vi "Tatica.vi"(9 "InfoMissao":T1 {"Agentes Disponíveis" format="%#_13g"}, 10 "test module 2":T2, 11 "IA State Input 2":T4 {"enemy_robots"."Agentes Disponíveis" format="%#_13g"; "our_robots"."Agentes Disponíveis" format="%#_13g"}) -> (1 "Robot 2":dbl(graph), 2 "ball 2":dbl(graph), 3 "IA State Output 2":T4 {"enemy_robots"."Agentes Disponíveis" format="%#_13g"; "our_robots"."Agentes Disponíveis" format="%#_13g"})   [LabVIEW 2018]
uses:
  Core/AI Input.ctl
  Core/AI Robot.ctl
  Intel/Functions Enum.ctl
  Intel/AttackerStates.ctl
  Path Planning/RRT/PathDests.ctl
  Path Planning/RRT/PathDest.ctl
  Core/AI Ball.ctl
  Core/Field Size.ctl
  Core/AI Judge.ctl
  Intel/Command Enum.ctl
  Util/Events/Events.ctl
  Test/TestModule.ctl
  Util/Select None or Robot.ctl
  InfoMissao.ctl
  <vilib>/Analysis/_algsub.llb/Real Vector Norm.vi
  <vilib>/Analysis/NI_AALPro.lvlib
panel:
  in  "test module":T2
  out "ball":dbl(graph)
  in  "atacando ao contrário?":bool=TRUE
  out "IA State Output":T4 {"enemy_robots"."Agentes Disponíveis" format="%#_13g"; "our_robots"."Agentes Disponíveis" format="%#_13g"}
  in  "IA State Input":T4 {"enemy_robots"."Agentes Disponíveis" format="%#_13g"; "our_robots"."Agentes Disponíveis" format="%#_13g"}
  out "Robot":dbl(graph)
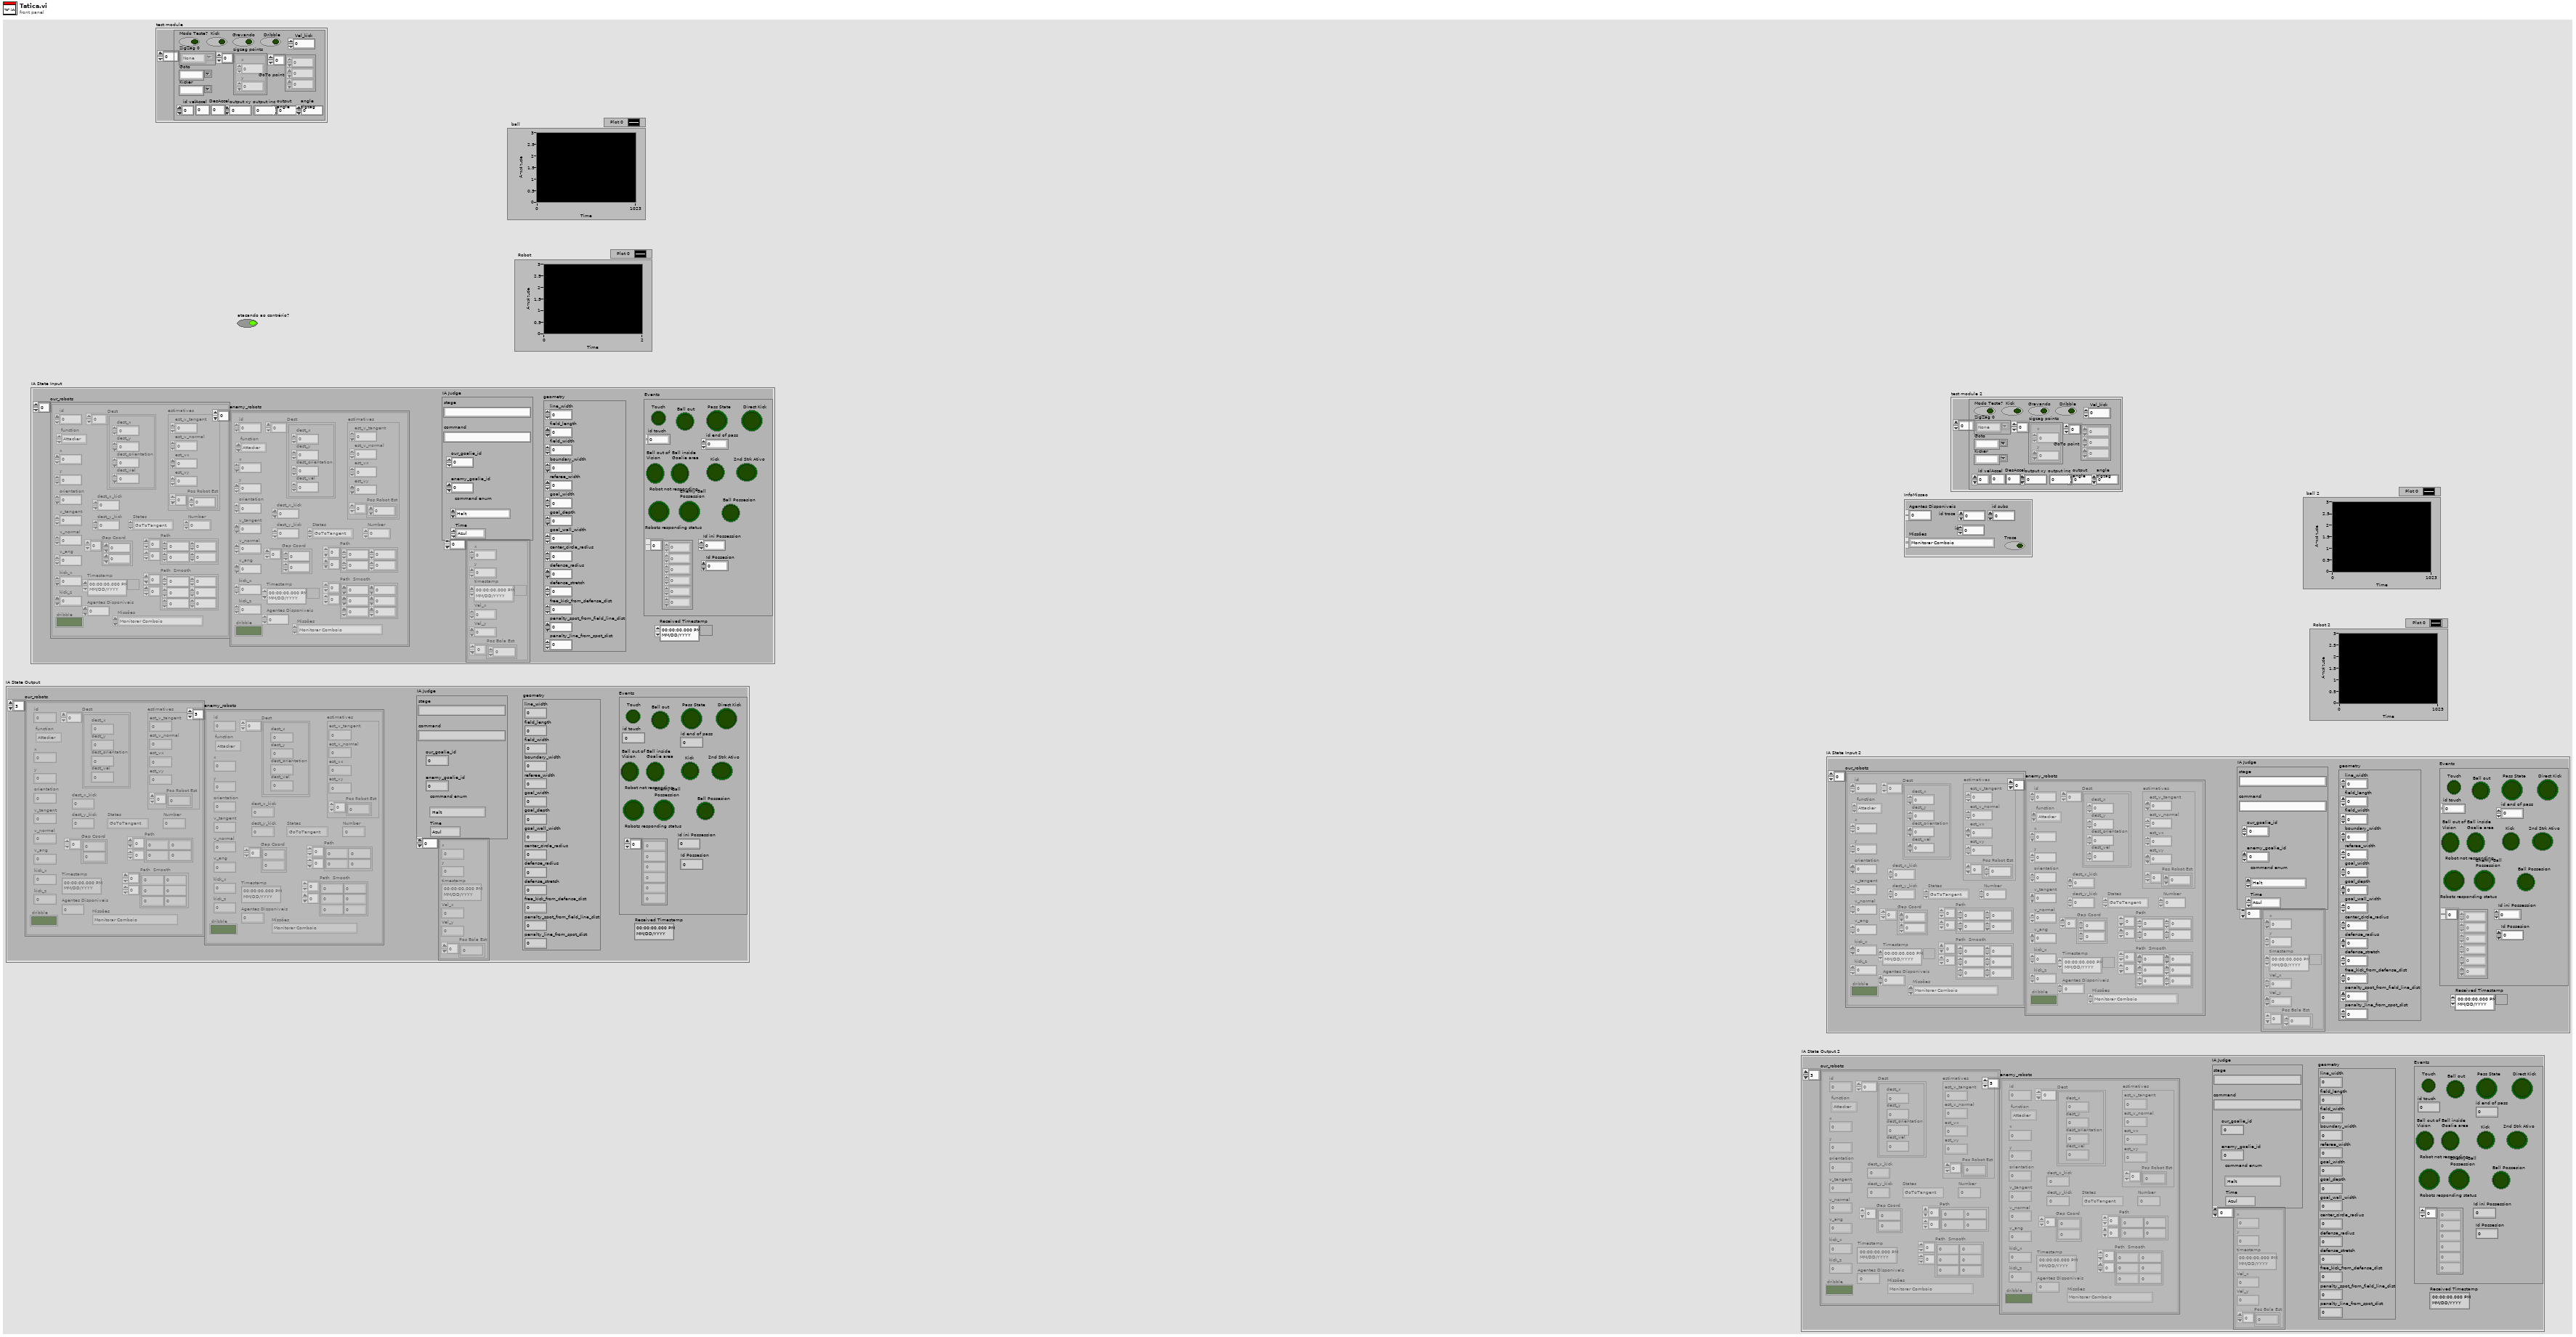
[diagram p1: front panel]
types:
  T1 = typedef "InfoMissao.ctl" = cluster{"Troca ":bool, "Missões ":enum16{"Monitorar Comboio", "Realizar Segurança de Retaguarda", "Vigiar Área", "Reconhecimento de Área"}, "Agentes Disponíveis":dbl, "id troca ":dbl, "id subs":dbl, "id ":dbl}
  T2 = typedef "TestModule.ctl" = cluster{"Goto":T3, "ZigZag 0":T3[], "Kicker":T3, "Vel_kick":dbl, "Kick":bool, "Modo Teste?":bool, "GoTo point":dbl[], "zigzag points":cluster{"x":dbl, "y":dbl}[], " id vel":u32, "Dribble":bool, "Gravando":bool, "output xy":dbl, "output\nangle":dbl, "angle\nzigzag":dbl, "output inc":dbl, "Accel":dbl, "DesAccel":dbl}
  T3 = typedef "Select None or Robot.ctl" = string
  T4 = typedef "AI Input.ctl" = cluster{"our_robots":T5[], "enemy_robots":T5[], "balls":T10[], "geometry":T11, "IA Judge":T12, "Received Timestamp":timestamp, "Events":T14}
  T5 = typedef "AI Robot.ctl" = cluster{"id":u32, "function":T6, "x":dbl, "y":dbl, "orientation":dbl, "v_tangent":dbl, "v_normal":dbl, "v_ang":dbl, "kick_x":dbl, "kick_z":dbl, "dribble":bool, "Timestamp":timestamp, "estimatives":cluster{"est_v_tangent":dbl, "est_v_normal":dbl, "est_vx":dbl, "est_vy":dbl, "Pos Robot Est":dbl[]}, "dest_x_kick":dbl, "dest_y_kick":dbl, "Gap Coord":dbl[], "States":T7, "Path ":dbl[][], "Path  Smooth":dbl[][], "Dest":T8, "Missões ":enum16{"Monitorar Comboio", "Realizar Segurança de Retaguarda", "Vigiar Área", "Reconhecimento de Área"}, "Agentes Disponíveis":dbl, "Number":dbl}
  T6 = typedef "Functions Enum.ctl" = enum16{"None", "Vigia", "2nd Striker", "Attacker", "Goalie", "Defender", "Striker", "Goto 0", "Dummy", "Kicker", "ZigZag 0", "ZigZag 1", "ZigZag 2", "ZigZag 3", "ZigZag 4", "ZigZag 5", "ZigZag 6", "ZigZag 7", "ZigZag 8", ""}
  T7 = typedef "AttackerStates.ctl" = enum16{"Pass", "GoToTangent", "BallGetting", "GoToKick", ""}
  T8 = typedef "PathDests.ctl" = T9[]
  T9 = typedef "PathDest.ctl" = cluster{"dest_x":dbl, "dest_y":dbl, "dest_orientation":dbl, "dest_vel":dbl}
  T10 = typedef "AI Ball.ctl" = cluster{"x":dbl, "y":dbl, "timestamp":timestamp, "Vel_x":dbl, "Vel_y":dbl, "Pos Bola Est":dbl[]}
  T11 = typedef "Field Size.ctl" = cluster{"line_width":u32, "field_length":u32, "field_width":u32, "boundary_width":u32, "referee_width":u32, "goal_width":u32, "goal_depth":u32, "goal_wall_width":u32, "center_circle_radius":u32, "defense_radius":u32, "defense_stretch":u32, "free_kick_from_defense_dist":u32, "penalty_spot_from_field_line_dist":u32, "penalty_line_from_spot_dist":u32}
  T12 = typedef "AI Judge.ctl" = cluster{"stage":string, "command":string, "our_goalie_id":dbl, "enemy_goalie_id":dbl, "command enum":T13, "Time":enum16{"Azul", "Amarelo"}}
  T13 = typedef "Command Enum.ctl" = enum16{"Halt", "Stop", "Force Start", "PKA Normal Start", "Prepare Kickoff Ally", "PKE Normal Start", "Prepare Kickoff Enemy", "Prepare Penalty Ally", "PPA Normal Start", "Prepare Penalty Enemy", "PPE Normal Start", "Direct Free Enemy", "Direct Free Ally", "Indirect Free Enemy", "Indirect Free Ally", "Timeout Enemy", "Timeout Ally", "Goal Enemy", "Goal Ally", "Ball Placement Enemy", "Ball Placement Ally", "Normal Half Time", "Extra Time Break", "Extra Half Time", "None", "Post Game"}
  T14 = typedef "Events.ctl" = cluster{"Touch":bool, "Ball out":bool, "id touch":dbl, "Ball out of \nVision":bool, "Ball inside \nGoalie area":bool, "Robot not responding":bool, "Robots responding status":dbl[], "Enemy Ball \nPossession":bool, "Pass State":bool, "id end of pass":dbl, "Kick":bool, "Id ini Possession":dbl, "Ball Possesion":bool, "Id Possesion":dbl, "Direct Kick":bool, "2nd Strk Ativo":bool}
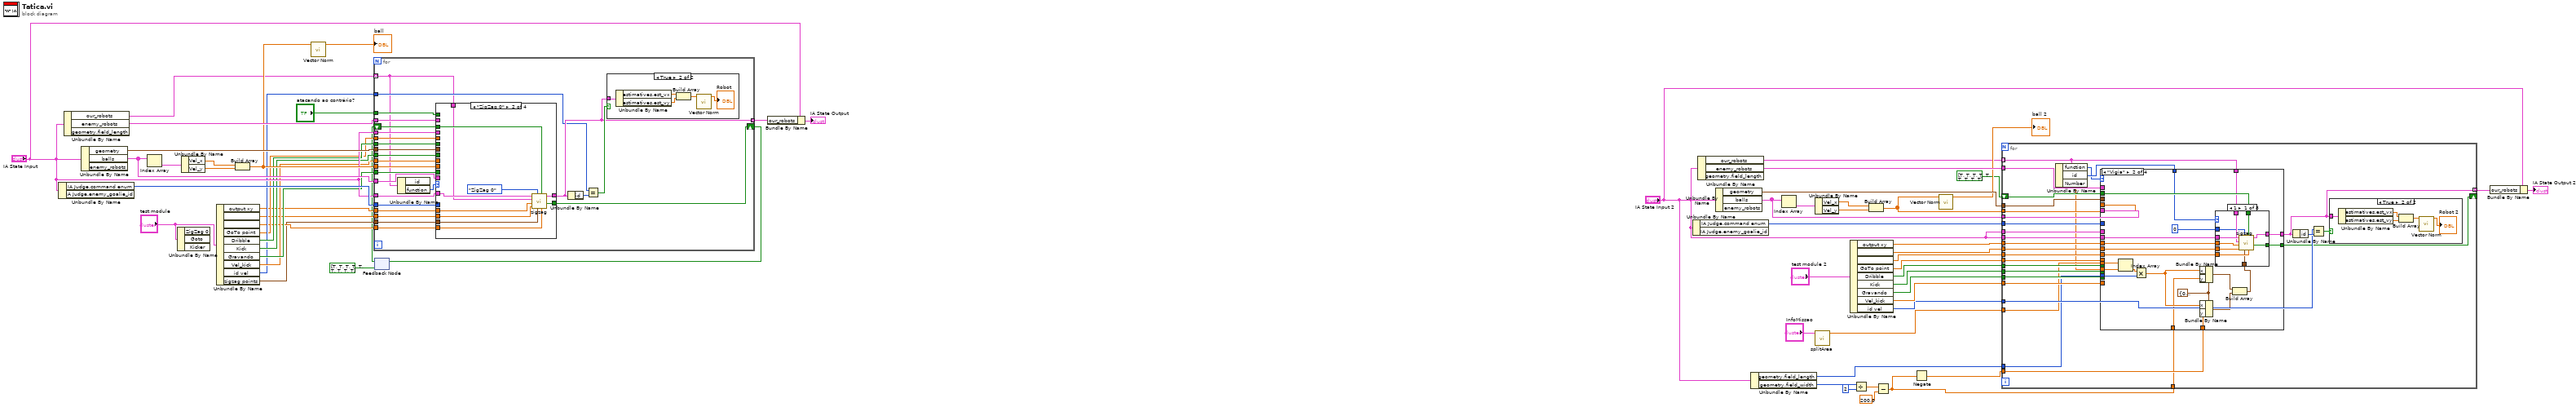
[diagram p0: block diagram]
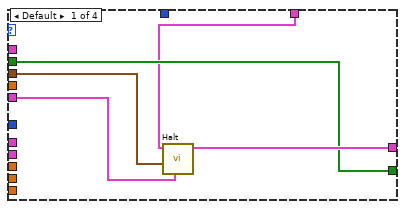
[diagram p3: hidden frame]
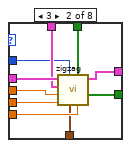
[diagram p4: hidden frame]
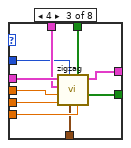
[diagram p5: hidden frame]
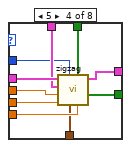
[diagram p6: hidden frame]
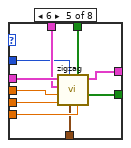
[diagram p7: hidden frame]
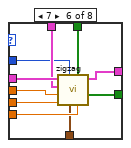
[diagram p8: hidden frame]
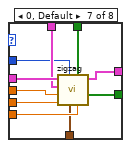
[diagram p9: hidden frame]
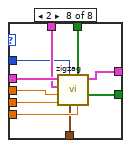
[diagram p10: hidden frame]
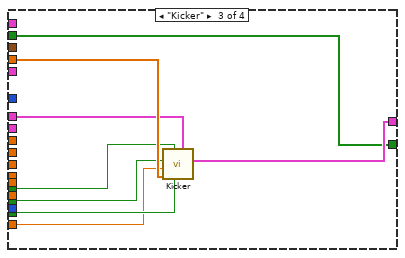
[diagram p11: hidden frame]
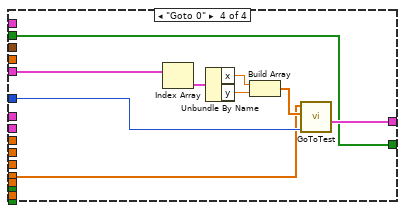
[diagram p12: hidden frame]
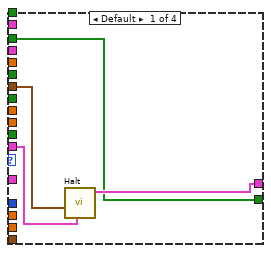
[diagram p14: hidden frame]
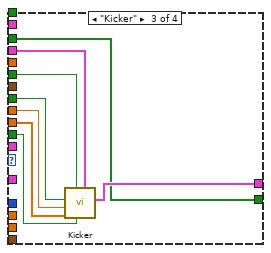
[diagram p15: hidden frame]
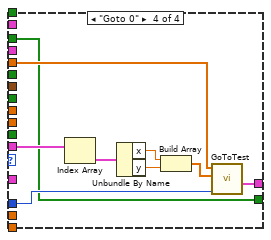
[diagram p16: hidden frame]
diagram:
  n1 = Unbundle By Name("IA State Input") -> ("IA Judge.command enum"=w61:T13)  [unwired: 1 out]
  n2 = Unbundle By Name("IA State Input") -> ("our_robots"=w6:T5[], "enemy_robots"=w57:T5[])  [unwired: 1 out]
  n3 = Unbundle By Name("IA State Input") -> ("geometry"=w58:T11, "balls"=w55:T10[])  [unwired: 1 out]
  n4 = Index Array(array=w55) -> (element=w54:T10)  [unwired: 1 in]
  n5 = Unbundle By Name("test module") -> ()  [unwired: 3 out]
  n6 = Unbundle By Name(w54) -> ("Vel_x"=w53:dbl, "Vel_y"=w52:dbl)
  n7 = Unbundle By Name("test module") -> ("output xy"=w41:dbl, "output\nangle"=w40:dbl, "angle\nzigzag"=w39:dbl, "GoTo point"=w42:dbl[], "Dribble"=w47:bool, "Kick"=w46:bool, "Gravando"=w45:bool, "Vel_kick"=w44:dbl, "id vel"=w43:u32, "zigzag points"=w38:cluster{"x":dbl, "y":dbl}[])
  n8 = Build Array(w53, w52) -> (w50:dbl[])
  n9 = call-poly <vilib>:"Vector Norm.vi"("Input Vector"=w50) -> ("norm"=→"ball":dbl)  [unwired: 9 in, 1 out]
  n10 = feedback #1(bool[] [TRUE, TRUE, TRUE, TRUE, TRUE, TRUE, TRUE, TRUE, TRUE]) -> (w35:bool[])
  n11 = for {
    tunnel: [w78] -> w60 mode=indexing
    tunnel: w61 -> [w86]
    tunnel: "IA State Input" -> [w85]
    tunnel: w58 -> [w84]
    tunnel: w55 -> [w83]
    tunnel: w57 -> [w82]
    tunnel: "atacando ao contrário?" -> [w81]
    tunnel: w38 -> [w77]
    tunnel: w50 -> [w76]
    tunnel: "IA State Input" -> [w75]
    tunnel: w47 -> [w74]
    tunnel: w46 -> [w73]
    tunnel: w45 -> [w72]
    tunnel: w44 -> [w71]
    tunnel: w43 -> [w70]
    tunnel: w42 -> [w69]
    tunnel: w41 -> [w68]
    tunnel: w40 -> [w67]
    tunnel: w39 -> [w66]
    shift-right: [w64] -> w37
    shift-left: w35 -> [w65]
    tunnel: w6 -> [w62] mode=indexing
    n12 = Unbundle By Name(w62) -> ("function"=w63:T6)  [unwired: 1 out]
    n13 = case shown="\"ZigZag 0\"" w63 {
      tunnel: [w95 w105 w113 w122] -> w78
      tunnel: w86 -> [_ _ _ w121]
      tunnel: w85 -> [_ w104 _ _]
      tunnel: w84 -> [w94 _ _ _]
      tunnel: w83 -> [w93 _ _ w120]
      tunnel: w82 -> [_ _ _ _]
      tunnel: w81 -> [_ _ _ _]
      tunnel: w77 -> [_ w103 _ _]
      tunnel: w76 -> [_ _ w112 _]
      tunnel: w75 -> [_ _ w111 _]
      tunnel: w74 -> [_ _ w110 _]
      tunnel: w73 -> [_ _ w109 _]
      tunnel: w72 -> [_ _ w108 _]
      tunnel: w71 -> [_ _ w107 _]
      tunnel: w69 -> [_ _ _ w115]
      tunnel: w68 -> [_ w102 _ _]
      tunnel: w67 -> [_ w101 _ _]
      tunnel: w66 -> [_ w100 _ _]
      tunnel: w65 -> [w92 w99 w106 w114]
      tunnel: [w92 w98 w106 w114] -> w64
      tunnel: w62 -> [_ w96 _ _]
      frame Default {
        n14 = call "Halt.vi"("balls"=w93, "Field Size in"=w94) -> ("Robot out"=w95:T5)  [unwired: 9 in]
      }
      frame "ZigZag 0" {
        n15 = call "zigzag.vi"("angulo"=w100, "Change point by ID"=w99, "points 3"=w103, "ZigZag Number"=Functions_Enum."ZigZag 0" ("y"), "output angle"=w101, "output xy"=w102, "Current Robot"=w96, "Al Input"=w104) -> ("output array"=w98:bool[], "Output Robot"=w105:T5)  [unwired: 1 in, 1 out]
      }
      frame "Kicker" {
        n16 = call "Kicker.vi"("IA State Input"=w111, "gravar"=w108, "Dribble"=w110, "Ball velocity"=w112, "Vel_kick"=w107, "Kick?"=w109) -> ("output cluster"=w113:T5)  [unwired: 5 in]
      }
      frame "Goto 0" {
        n17 = Index Array(array=w120) -> (element=w119:T10)  [unwired: 1 in]
        n18 = Unbundle By Name(w119) -> ("x"=w118:dbl, "y"=w117:dbl)
        n19 = Build Array(w118, w117) -> (w116:dbl[])
        n20 = call "GoToTest.vi"("command\nenum"=w121, "Ball"=w116, "GoTo point"=w115) -> ("Robot Out"=w122:T5)  [unwired: 8 in]
      }
    }
    n21 = Unbundle By Name(w78) -> ("id"=w80:u32)
    n22 = Equal?(x=w70, y=w80) -> (x = y?=w79:bool)
    n23 = case shown="True" w79 {
      tunnel: w78 -> [_ w91]
      frame False {
      }
      frame True {
        n24 = Unbundle By Name(w91) -> ("estimatives.est_vx"=w90:dbl, "estimatives.est_vy"=w89:dbl)
        n25 = Build Array(w90, w89) -> (w88:dbl[])
        n26 = call-poly <vilib>:"Vector Norm.vi"("Input Vector"=w88) -> ("norm"=→"Robot":dbl)  [unwired: 9 in, 1 out]
      }
    }
  }
  n27 = feedback-in #1(w37) -> ()
  n28 = Bundle By Name(cluster="IA State Input", "our_robots"=w60) -> (→"IA State Output":T4)
  n29 = Unbundle By Name("IA State Input 2") -> ("IA Judge.command enum"=w34:T13)  [unwired: 1 out]
  n30 = Unbundle By Name("IA State Input 2") -> ("our_robots"=w13:T5[], "enemy_robots"=w30:T5[])  [unwired: 1 out]
  n31 = Unbundle By Name("IA State Input 2") -> ("geometry"=w31:T11, "balls"=w29:T10[])  [unwired: 1 out]
  n32 = Unbundle By Name("IA State Input 2") -> ("geometry.field_length"=w3:u32, "geometry.field_width"=w10:u32)
  n33 = Index Array(array=w29) -> (element=w28:T10)  [unwired: 1 in]
  n34 = call "splitArea.vi"("InfoMissao"="InfoMissao") -> ("Array"=w4:dbl[])  [unwired: 10 in]
  n35 = Unbundle By Name(w28) -> ("Vel_x"=w27:dbl, "Vel_y"=w26:dbl)
  n36 = Unbundle By Name("test module 2") -> ("output xy"=w16:dbl, "output\nangle"=w15:dbl, "angle\nzigzag"=w14:dbl, "GoTo point"=w17:dbl[], "Dribble"=w22:bool, "Kick"=w21:bool, "Gravando"=w20:bool, "Vel_kick"=w19:dbl, "id vel"=w18:u32)
  n37 = Divide(x=w10, y=u32 2) -> (x/y=w8:dbl)
  n38 = Build Array(w27, w26) -> (w24:dbl[])
  n39 = Subtract(x=w8, y=200.0) -> (x-y=w1:dbl)
  n40 = Negate(x=w1) -> (-x=w2:dbl)
  n41 = call-poly <vilib>:"Vector Norm.vi"("Input Vector"=w24) -> ("norm"=→"ball 2":dbl)  [unwired: 9 in, 1 out]
  n42 = for {
    tunnel: [w144] -> w33 mode=indexing
    tunnel: w34 -> [w151]
    tunnel: "IA State Input 2" -> [w150]
    tunnel: w31 -> [w149]
    tunnel: w29 -> [w148]
    tunnel: w30 -> [w147]
    tunnel: w24 -> [w143]
    tunnel: "IA State Input 2" -> [w142]
    tunnel: w22 -> [w141]
    tunnel: w21 -> [w140]
    tunnel: w20 -> [w139]
    tunnel: w19 -> [w138]
    tunnel: w18 -> [w137]
    tunnel: w17 -> [w136]
    tunnel: w16 -> [w135]
    tunnel: w15 -> [w134]
    tunnel: w14 -> [w133]
    shift-right: [w131] -> _
    shift-left: bool[] [TRUE, TRUE, TRUE, TRUE, TRUE, TRUE, TRUE, TRUE, TRUE] -> [w132]
    tunnel: w13 -> [w130] mode=indexing
    tunnel: w4 -> [w128]
    tunnel: w3 -> [w126]
    tunnel: w2 -> [w125]
    tunnel: w1 -> [w124]
    n43 = Unbundle By Name(w130) -> ("function"=w123:T6, "id"=w129:u32, "Number"=w127:dbl)
    n44 = case shown="\"Vigia\"" w123 {
      tunnel: [w161 w182 w270 w279] -> w144
      tunnel: w151 -> [_ _ _ w278]
      tunnel: w150 -> [_ w181 _ _]
      tunnel: w149 -> [w160 _ _ _]
      tunnel: w148 -> [w159 _ _ w277]
      tunnel: w147 -> [_ _ _ _]
      tunnel: w143 -> [_ _ w269 _]
      tunnel: w142 -> [_ _ w268 _]
      tunnel: w141 -> [_ _ w267 _]
      tunnel: w140 -> [_ _ w266 _]
      tunnel: w139 -> [_ _ w265 _]
      tunnel: w138 -> [_ _ w264 _]
      tunnel: w136 -> [_ _ _ w272]
      tunnel: w135 -> [_ w180 _ _]
      tunnel: w134 -> [_ w179 _ _]
      tunnel: w133 -> [_ w178 _ _]
      tunnel: w132 -> [w158 w177 w263 w271]
      tunnel: [w158 w176 w263 w271] -> w131
      tunnel: w130 -> [w157 w175 _ _]
      tunnel: w129 -> [_ w173 _ _]
      tunnel: w128 -> [_ w168 _ _]
      tunnel: w127 -> [_ w167 _ _]
      tunnel: w126 -> [_ w166 _ _]
      tunnel: w125 -> [_ w164 _ _]
      tunnel: w124 -> [_ w163 _ _]
      frame Default {
        n45 = call "Halt.vi"("balls"=w159, "Field Size in"=w160, "Robot in"=w157) -> ("Robot out"=w161:T5)  [unwired: 8 in]
      }
      frame "Vigia" {
        w165 = cluster{"x":dbl, "y":dbl} {"x"=0.0, "y"=0.0} ("element")
        n46 = Index Array(array=w168, index=w167) -> (element=w172:dbl)
        n47 = Multiply(x=w172, y=w166) -> (x*y=w171:dbl)
        n48 = Bundle By Name(cluster=w165, "x"=w171, "y"=w163) -> (w169:cluster{"x":dbl, "y":dbl})
        n49 = Bundle By Name(cluster=w165, "x"=w171, "y"=w164) -> (w170:cluster{"x":dbl, "y":dbl})
        n50 = Build Array(w169, w170) -> (w162:cluster{"x":dbl, "y":dbl}[])
        n51 = case shown="1" w173 {
          tunnel: [w192 w202 w212 w222 w232 w242 w252 w262] -> w182
          tunnel: w181 -> [w191 w201 w211 w221 w231 w241 w251 w261]
          tunnel: w180 -> [w190 w200 w210 w220 w230 w240 w250 w260]
          tunnel: w179 -> [w189 w199 w209 w219 w229 w239 w249 w259]
          tunnel: w178 -> [w188 w198 w208 w218 w228 w238 w248 w258]
          tunnel: w177 -> [w187 w197 w207 w217 w227 w237 w247 w257]
          tunnel: [w186 w196 w206 w216 w226 w236 w246 w256] -> w176
          tunnel: w175 -> [w185 w195 w205 w215 w225 w235 w245 w255]
          tunnel: w162 -> [w184 w194 w204 w214 w224 w234 w244 w254]
          tunnel: u16 0 ("ZigZag Number") -> [w183 w193 w203 w213 w223 w233 w243 w253]
          frame 1 {
            n52 = call "zigzag.vi"("angulo"=w188, "Change point by ID"=w187, "points 3"=w184, "ZigZag Number"=w183, "output angle"=w189, "output xy"=w190, "Current Robot"=w185, "Al Input"=w191) -> ("output array"=w186:bool[], "Output Robot"=w192:T5)  [unwired: 1 in, 1 out]
          }
          frame 3 {
            n53 = call "zigzag.vi"("angulo"=w198, "Change point by ID"=w197, "points 3"=w194, "ZigZag Number"=w193, "output angle"=w199, "output xy"=w200, "Current Robot"=w195, "Al Input"=w201) -> ("output array"=w196:bool[], "Output Robot"=w202:T5)  [unwired: 1 in, 1 out]
          }
          frame 4 {
            n54 = call "zigzag.vi"("angulo"=w208, "Change point by ID"=w207, "points 3"=w204, "ZigZag Number"=w203, "output angle"=w209, "output xy"=w210, "Current Robot"=w205, "Al Input"=w211) -> ("output array"=w206:bool[], "Output Robot"=w212:T5)  [unwired: 1 in, 1 out]
          }
          frame 5 {
            n55 = call "zigzag.vi"("angulo"=w218, "Change point by ID"=w217, "points 3"=w214, "ZigZag Number"=w213, "output angle"=w219, "output xy"=w220, "Current Robot"=w215, "Al Input"=w221) -> ("output array"=w216:bool[], "Output Robot"=w222:T5)  [unwired: 1 in, 1 out]
          }
          frame 6 {
            n56 = call "zigzag.vi"("angulo"=w228, "Change point by ID"=w227, "points 3"=w224, "ZigZag Number"=w223, "output angle"=w229, "output xy"=w230, "Current Robot"=w225, "Al Input"=w231) -> ("output array"=w226:bool[], "Output Robot"=w232:T5)  [unwired: 1 in, 1 out]
          }
          frame 7 {
            n57 = call "zigzag.vi"("angulo"=w238, "Change point by ID"=w237, "points 3"=w234, "ZigZag Number"=w233, "output angle"=w239, "output xy"=w240, "Current Robot"=w235, "Al Input"=w241) -> ("output array"=w236:bool[], "Output Robot"=w242:T5)  [unwired: 1 in, 1 out]
          }
          frame 0, Default {
            n58 = call "zigzag.vi"("angulo"=w248, "Change point by ID"=w247, "points 3"=w244, "ZigZag Number"=w243, "output angle"=w249, "output xy"=w250, "Current Robot"=w245, "Al Input"=w251) -> ("output array"=w246:bool[], "Output Robot"=w252:T5)  [unwired: 1 in, 1 out]
          }
          frame 2 {
            n59 = call "zigzag.vi"("angulo"=w258, "Change point by ID"=w257, "points 3"=w254, "ZigZag Number"=w253, "output angle"=w259, "output xy"=w260, "Current Robot"=w255, "Al Input"=w261) -> ("output array"=w256:bool[], "Output Robot"=w262:T5)  [unwired: 1 in, 1 out]
          }
        }
      }
      frame "Kicker" {
        n60 = call "Kicker.vi"("IA State Input"=w268, "gravar"=w265, "Dribble"=w267, "Ball velocity"=w269, "Vel_kick"=w264, "Kick?"=w266) -> ("output cluster"=w270:T5)  [unwired: 5 in]
      }
      frame "Goto 0" {
        n61 = Index Array(array=w277) -> (element=w276:T10)  [unwired: 1 in]
        n62 = Unbundle By Name(w276) -> ("x"=w275:dbl, "y"=w274:dbl)
        n63 = Build Array(w275, w274) -> (w273:dbl[])
        n64 = call "GoToTest.vi"("command\nenum"=w278, "Ball"=w273, "GoTo point"=w272) -> ("Robot Out"=w279:T5)  [unwired: 8 in]
      }
    }
    n65 = Unbundle By Name(w144) -> ("id"=w146:u32)
    n66 = Equal?(x=w137, y=w146) -> (x = y?=w145:bool)
    n67 = case shown="True" w145 {
      tunnel: w144 -> [_ w156]
      frame False {
      }
      frame True {
        n68 = Unbundle By Name(w156) -> ("estimatives.est_vx"=w155:dbl, "estimatives.est_vy"=w154:dbl)
        n69 = Build Array(w155, w154) -> (w153:dbl[])
        n70 = call-poly <vilib>:"Vector Norm.vi"("Input Vector"=w153) -> ("norm"=→"Robot 2":dbl)  [unwired: 9 in, 1 out]
      }
    }
  }
  n71 = Bundle By Name(cluster="IA State Input 2", "our_robots"=w33) -> (→"IA State Output 2":T4)
